vi "Parse Request.vi"(8 "error in (no error)":errorcluster, 10 "{JSON} Request":string, 11 "JSON-RPC in":refnum<class "JSON-RPC.lvclass">) -> (0 "error out":errorcluster, 1 "Params":string[](array[string]), 2 "Methods":string[](array[string]), 3 "JSON-RPC out":refnum<class "JSON-RPC.lvclass">)   [LabVIEW 2019, in "JSON-RPC.lvclass"]
uses:
  JSON-RPC.lvclass
  JSON-RPC.lvclass/JSON-RPC.ctl
  private/Parse Request-JSONtext.vi/523bbeac-5bfa-4355-a479-ec0e355c2dae.vi
  private/Parse Request-JSONtext.vi/5dfc14ef-dff6-4e36-b5f1-09fb62becacc.vi
  private/Parse Request-JSONtext.vi/f339b867-7010-45a6-b71e-b2a9da4366e1.vi
  <vilib>/JDP Science/JSONtext/Find Item.vi
  <vilib>/JDP Science/JSONtext/String Subset.vi
  <vilib>/JDP Science/JSONtext/Get all Object Items.vi
  <vilib>/JDP Science/JSONtext/Parsing/Parse Full Path or Item Name.vi
  <vilib>/JDP Science/JSONtext/Next JSON Value.vi
  <vilib>/JDP Science/JSONtext/support/Error Cluster From Code.vi
  <vilib>/JDP Science/JSONtext/Offset/Find Item Locations by Path.vi
  <vilib>/JDP Science/JSONtext/JSON text to Variant.vi
  <vilib>/JDP Science/JSONtext/LVClass Serializer/JSONtext LVClass Serializer.lvclass
  <vilib>/JDP Science/JSONtext/JSONtext.lvlib
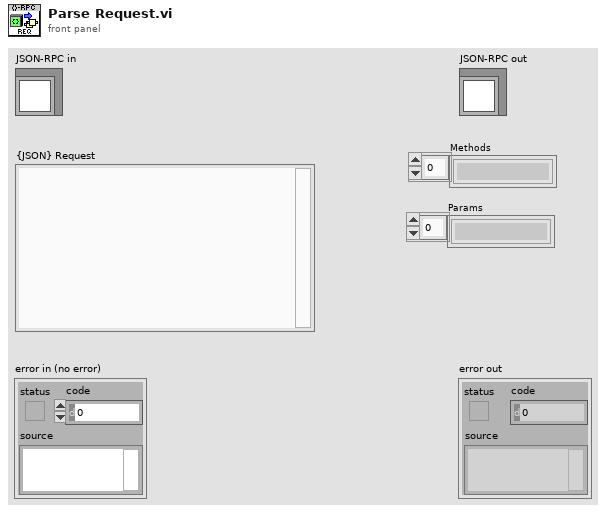
[diagram p1: front panel]
types:
  T1 = typedef "JSONtext.lvlib/JSON Value Type.ctl" = enum16{"Not a JSON Value", "JSON Object", "JSON Array", "String", "Number", "true", "false", "null"}
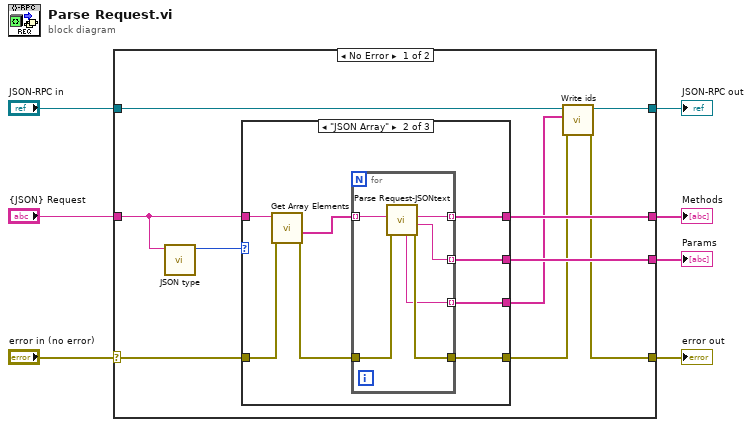
[diagram p0: block diagram]
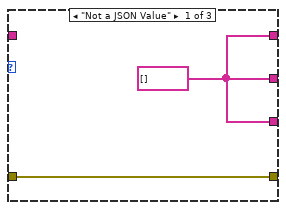
[diagram p2: hidden frame]
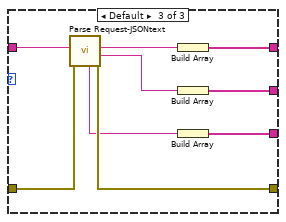
[diagram p3: hidden frame]
diagram:
  n1 = case shown="No Error" "error in (no error)" {
    selector: "error in (no error)" -> [w14 w44]
    tunnel: [w10 w44] -> w6
    tunnel: [w9 w43] -> w4
    tunnel: "JSON-RPC in" -> [w8 w43]
    tunnel: "{JSON} Request" -> [w13 _]
    tunnel: [w17 _] -> w1
    tunnel: [w16 _] -> w2
    frame No Error {
      n2 = call <vilib>:"JSON type.vi"("JSON"=w13) -> ("JSON Value Type"=w15:T1)  [unwired: 9 in, 1 out]
      n3 = case shown="\"JSON Array\"" w15 {
        tunnel: w14 -> [w19 w23 w37]
        tunnel: [w19 w27 w36] -> w11
        tunnel: w13 -> [_ w24 w40]
        tunnel: [w18 w26 w42] -> w16
        tunnel: [w18 w25 w41] -> w17
        tunnel: [w18 w21 w34] -> w12
        frame "Not a JSON Value" {
          w18 = string[] []
        }
        frame "JSON Array" {
          n4 = call <vilib>:"Get Array Elements.vi"("error in (no error)"=w23, "JSON"=w24) -> ("error out"=w20:errorcluster, "<JSON>"=w22:string[])  [unwired: 7 in, 1 out]
          n5 = for {
            tunnel: w22 -> [w31] mode=indexing
            tunnel: [w30] -> w26 mode=indexing
            tunnel: [w28] -> w25 mode=indexing
            tunnel: [w29] -> w21 mode=indexing
            tunnel: w20 -> [w32]
            tunnel: [w33] -> w27
            n6 = call "Parse Request-JSONtext.vi"("error in (no error)"=w32, "{JSON} Request"=w31) -> ("error out"=w33:errorcluster, "params"=w28:string, "method"=w30:string, "id"=w29:string)  [unwired: 6 in]
          }
        }
        frame Default {
          n7 = call "Parse Request-JSONtext.vi"("error in (no error)"=w37, "{JSON} Request"=w40) -> ("error out"=w36:errorcluster, "params"=w38:string, "method"=w39:string, "id"=w35:string)  [unwired: 6 in]
          n8 = Build Array(w39) -> (w42:string[])
          n9 = Build Array(w38) -> (w41:string[])
          n10 = Build Array(w35) -> (w34:string[])
        }
      }
      n11 = call "Write ids.vi"("error in (no error)"=w11, "ids"=w12, "JSON-RPC in"=w8) -> ("error out"=w10:errorcluster, "JSON-RPC out"=w9:refnum<class "JSON-RPC.lvclass">)  [unwired: 7 in]
    }
    frame Error {
    }
  }
  "error out" <- w6
  "JSON-RPC out" <- w4
  "Methods" <- w2
  "Params" <- w1
